vi "未命名 1.vi"() -> ()   [LabVIEW 2014]
uses:
  <vilib>/vision/NI_Vision_Development_Module.lvlib
panel:
  out "Image":T1(plugin-control)
  in  "Structuring Element":i32[][](array[numeric])=[[1, 1, 1], [1, 1, 1], [1, 1, 1]]
  in  "Operation":T2(ring)
  in  "Number of Erosion":i32=2
  out "Image 2":T1(plugin-control)
  out "Histogram":T3(graph)
  out "Standard Deviation":sgl format="%#.2f"
  out "Mean":sgl format="%#.2f"
  in  "Stop":bool
  in  "Range":cluster{"Lower value":sgl, "Upper value":sgl}={"Lower value"=128.0, "Upper value"=255.0} {"Upper value" format="%.2f"; "Lower value" format="%.2f"}
  in  "File Path":path
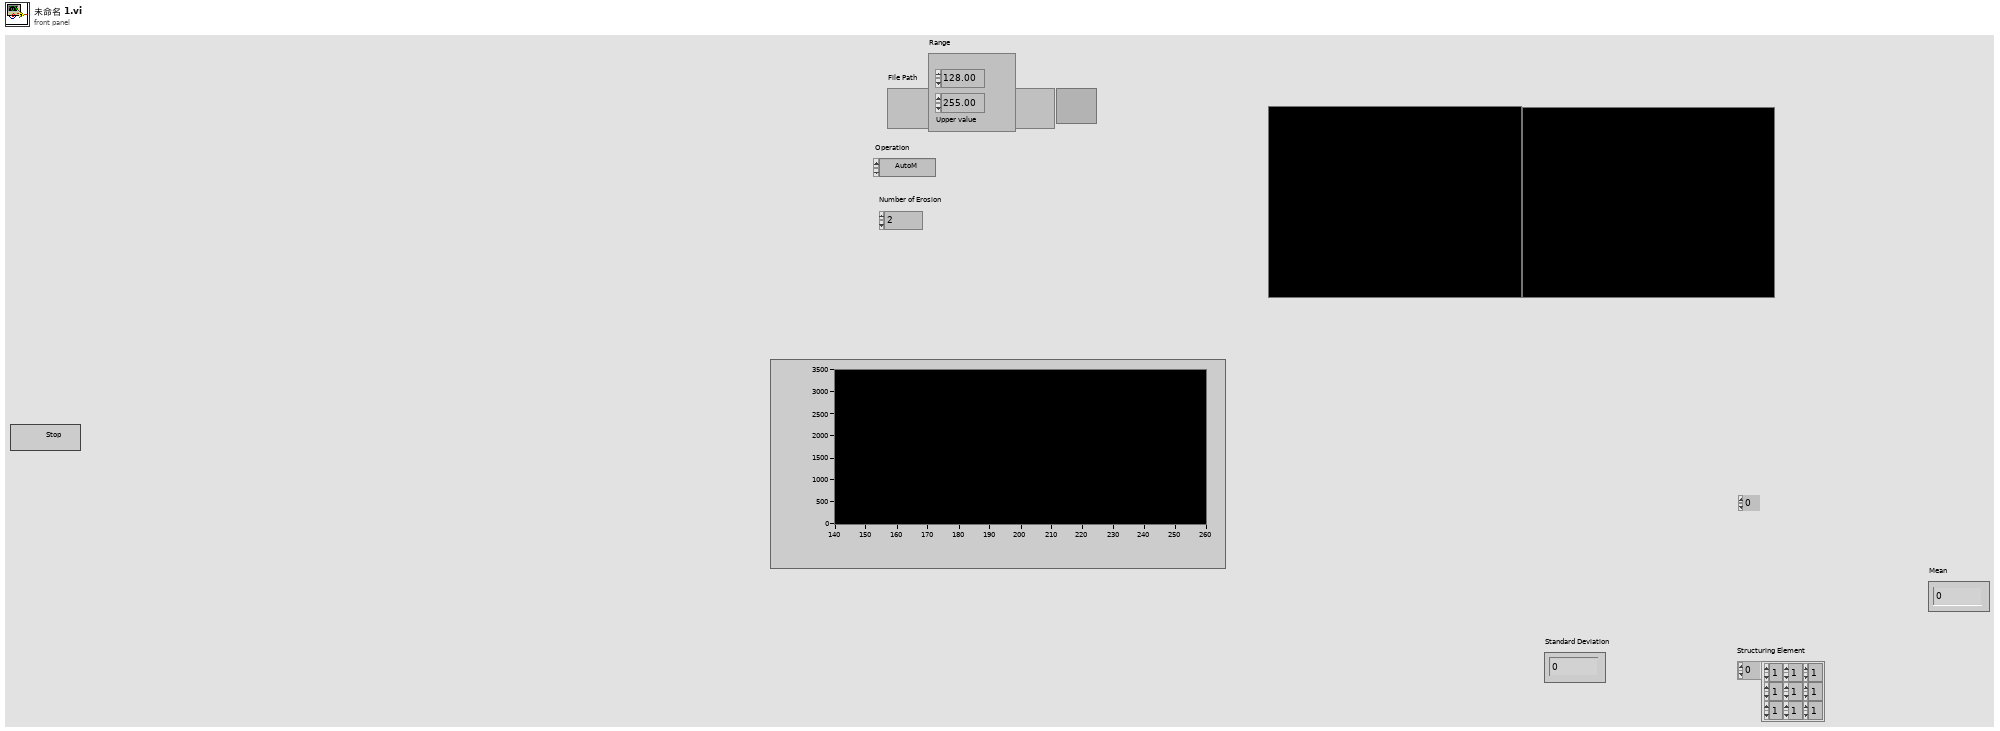
[diagram p1: front panel]
types:
  T1 = typedef "IMAQ Image.ctl" = refnum<image>
  T2 = enum32{"AutoM", "Close", "Dilate", "Erode", "Gradient", "Gradient out", "Gradient in", "Hit miss", "Open", "PClose", "POpen", "Thick", "Thin"}
  T3 = cluster{"Starting Value":sgl, "Incremental Value":sgl, "Histogram":u32[]}
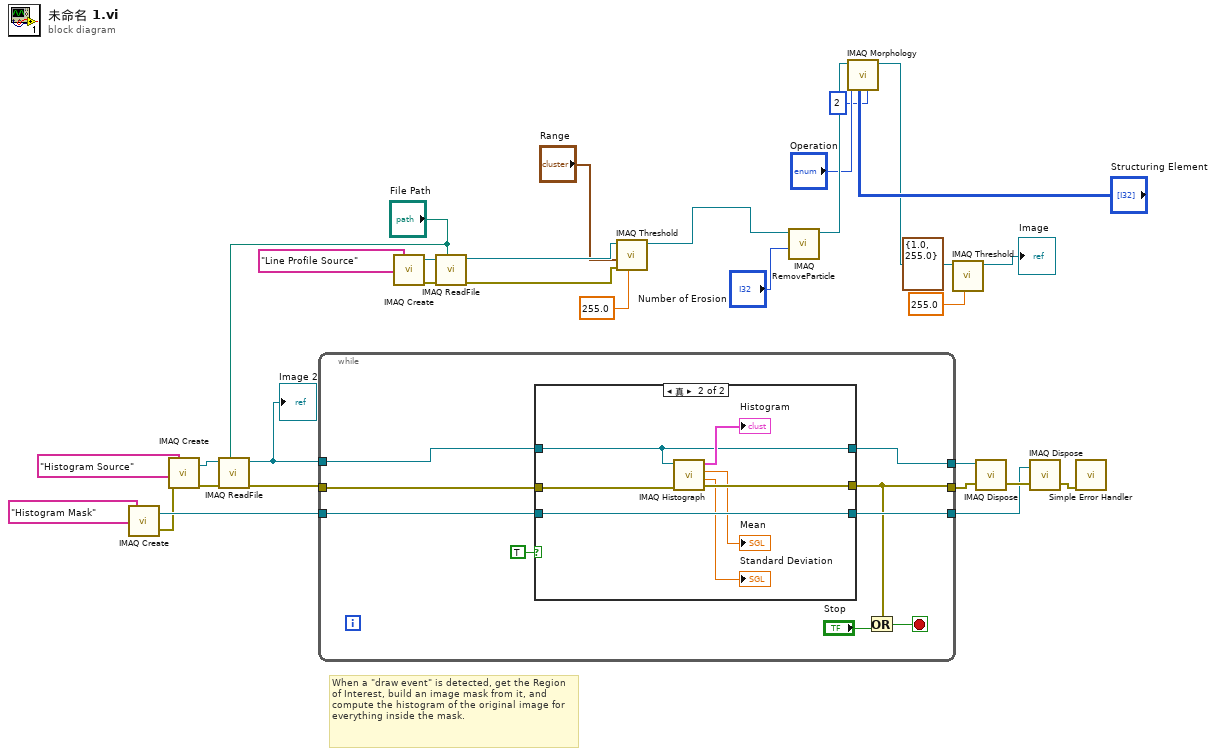
[diagram p0: block diagram]
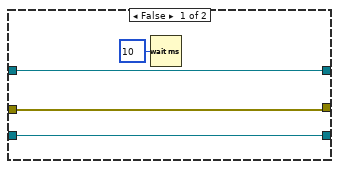
[diagram p2: hidden frame]
diagram:
  # "When a \"draw event\" is detected, get the Region of Interest, build an image mask from it, and compute the histogram of the original image for everything inside the mask."
  n1 = call "IMAQ Create"("Image Name"="Histogram Mask") -> ("New Image"=w20:T1, "error out"=w14:errorcluster)  [unwired: 4 in]
  n2 = call "IMAQ Create"("Image Name"="Histogram Source", "error in (no error)"=w14) -> ("New Image"=w25:T1, "error out"=w24:errorcluster)  [unwired: 3 in]
  n3 = call "IMAQ ReadFile"("File Path"="File Path", "error in (no error)"=w24, "Image"=w25) -> ("error out"=w22:errorcluster, "Image Out"=w13:T1)  [unwired: 4 in, 3 out]
  "Image 2" <- w13
  n4 = while {
    tunnel: w13 -> [w32]
    tunnel: w22 -> [w35]
    tunnel: w20 -> [w36]
    tunnel: [w34] -> w19
    tunnel: [w39] -> w15
    tunnel: [w38] -> w16
    stop <- w37 stop-if-true
    n5 = case shown="真" TRUE {
      tunnel: w32 -> [w43 w48]
      tunnel: w36 -> [w42 w49]
      tunnel: [w41 w51] -> w34
      tunnel: [w42 w49] -> w39
      tunnel: [w43 w48] -> w38
      tunnel: w35 -> [w41 w45]
      frame False {
        n6 = Wait (ms)(milliseconds to wait=u32 10) -> ()  [unwired: 1 out]
      }
      frame True {
        n7 = call "IMAQ Histograph"("error in (no error)"=w45, "Image"=w48) -> ("error out"=w51:errorcluster, "Standard  Deviation"=→"Standard Deviation":sgl, "Mean Value"=→"Mean":sgl, "Histogram Graph"=→"Histogram":T3)  [unwired: 6 in]
      }
    }
    n8 = Or(x=w34, y="Stop") -> (x .or. y?=w37:bool)
  }
  n9 = call "IMAQ Create"("Image Name"="Line Profile Source") -> ("New Image"=w31:T1, "error out"=w30:errorcluster)  [unwired: 4 in]
  n10 = call "IMAQ ReadFile"("File Path"="File Path", "error in (no error)"=w30, "Image"=w31) -> ("error out"=w28:errorcluster, "Image Out"=w27:T1)  [unwired: 4 in, 3 out]
  n11 = call "IMAQ Threshold"("Replace Value"=sgl 255.0, "error in (no error)"=w28, "Range"="Range", "Image Src"=w27) -> ("Image Dst Out"=w11:T1)  [unwired: 2 in, 5 out]
  n12 = call "IMAQ RemoveParticle"("Number of Erosion"="Number of Erosion", "Image Src"=w11) -> ("Image Dst Out"=w8:T1)  [unwired: 8 in, 1 out]
  n13 = call "IMAQ Morphology"("Number of iterations (1)"=2, "Structuring Element"="Structuring Element", "Operation"="Operation", "Image Src"=w8) -> ("Image Dst Out"=w5:T1)  [unwired: 6 in, 1 out]
  n14 = call "IMAQ Threshold"("Replace Value"=sgl 255.0, "Range"=cluster{"Lower value":sgl, "Upper value":sgl} {"Lower value"=1.0, "Upper value"=255.0}, "Image Src"=w5) -> ("Image Dst Out"=→"Image":T1)  [unwired: 3 in, 5 out]
  n15 = call "IMAQ Dispose"("Image"=w16, "error in (no error)"=w19) -> ("error out"=w18:errorcluster)  [unwired: 4 in]
  n16 = call "IMAQ Dispose"("Image"=w15, "error in (no error)"=w18) -> ("error out"=w17:errorcluster)  [unwired: 4 in]
  n17 = call <vilib>:"Simple Error Handler.vi"("error in (no error)"=w17) -> ()  [unwired: 4 in, 5 out]
